vi "Get Random Piece Index.vi"(8 "error in (no error)":errorcluster caption="entrée d'erreur (pas d'erreur)") -> (0 "error out":errorcluster caption="sortie d'erreur", 3 "Piece index":u16)   [LabVIEW 2017]
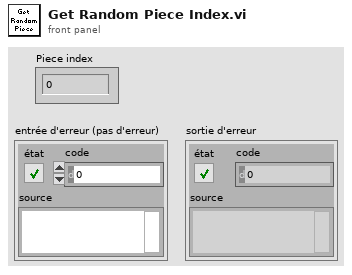
[diagram p1: front panel]
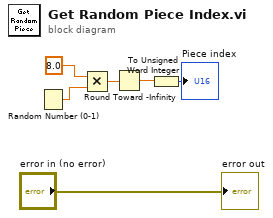
[diagram p0: block diagram]
diagram:
  n1 = Random Number (0-1)() -> (number: 0 to 1=w2:dbl)
  n2 = Multiply(x=8.0, y=w2) -> (x*y=w4:dbl)
  n3 = Round Toward -Infinity(1:w4) -> (0:w5:dbl)
  n4 = To Unsigned Word Integer(number=w5) -> (unsigned 16bit integer=→"Piece index":u16)
  "error out" <- "error in (no error)"
